vi "Check_Single_Box_move.vi"(3 "Traverse Name":string, 5 "Exclude Array":T3[](array[typedef])=[{"Sizes"=[{"Max"=15000.0, "Min"=0.0}, {"Max"=1000.0, "Min"=-1000.0}, {"Max"=300.0, "Min"=0.0}], "Name"="Roughness Elements", "Exclude Type"=enum."Allow only vertical moves"}, {"Sizes"=[{"Max"=17000.0, "Min"=16000.0}, {"Max"=200.0, "Min"=-200.0}, {"Max"=-50.0, "Min"=-250.0}], "Name"="B204", "Exclude Type"=enum."Exclude completely"}] {"Sizes"."Min" format="%#.1f"; "Sizes"."Max" format="%#.1f"}, 6 "Volume":T2=[{"Max"=15001.0, "Min"=12000.0}, {"Max"=1000.0, "Min"=-1000.0}, {"Max"=700.0, "Min"=0.0}] {"Min" format="%#.1f"; "Max" format="%#.1f"}, 8 "New Position":sgl[](array[numeric])=[0.0, 0.0, 0.0] format="%.2f", 9 "Current position":sgl[](array[numeric])=[0.0, 0.0, 0.0] format="%.2f") -> (0 "Error Comments":string, 2 "Position At Crash":dbl[](array[numeric]) format="%.2f")   [LabVIEW 2018]
uses:
  Exclude_cluster.ctl
  Box_size.ctl
  Exclusion_type.ctl
  Moving Axis.ctl
  Globals/Trav_pos_global.vi
panel:
  in  "Traverse active parts":T1
  out "Numeric":i32
  # "X                Y                   Z"
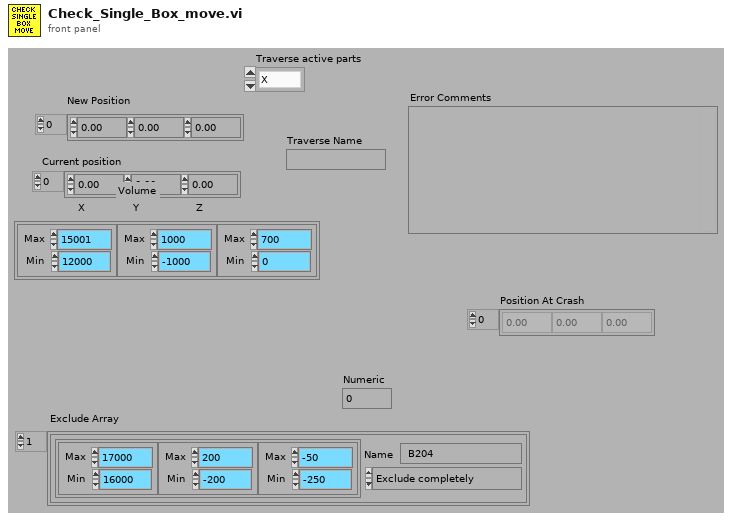
[diagram p1: front panel]
types:
  T1 = typedef "Moving Axis.ctl" = enum16{"X", "XY", "XYZ"}
  T2 = typedef "Box_size.ctl" = cluster{"Max":sgl, "Min":sgl}[]
  T3 = typedef "Exclude_cluster.ctl" = cluster{"Sizes":T2, "Name":string, "Exclude Type":T4}
  T4 = typedef "Exclusion_type.ctl" = enum16{"Exclude completely", "Allow only vertical moves"}
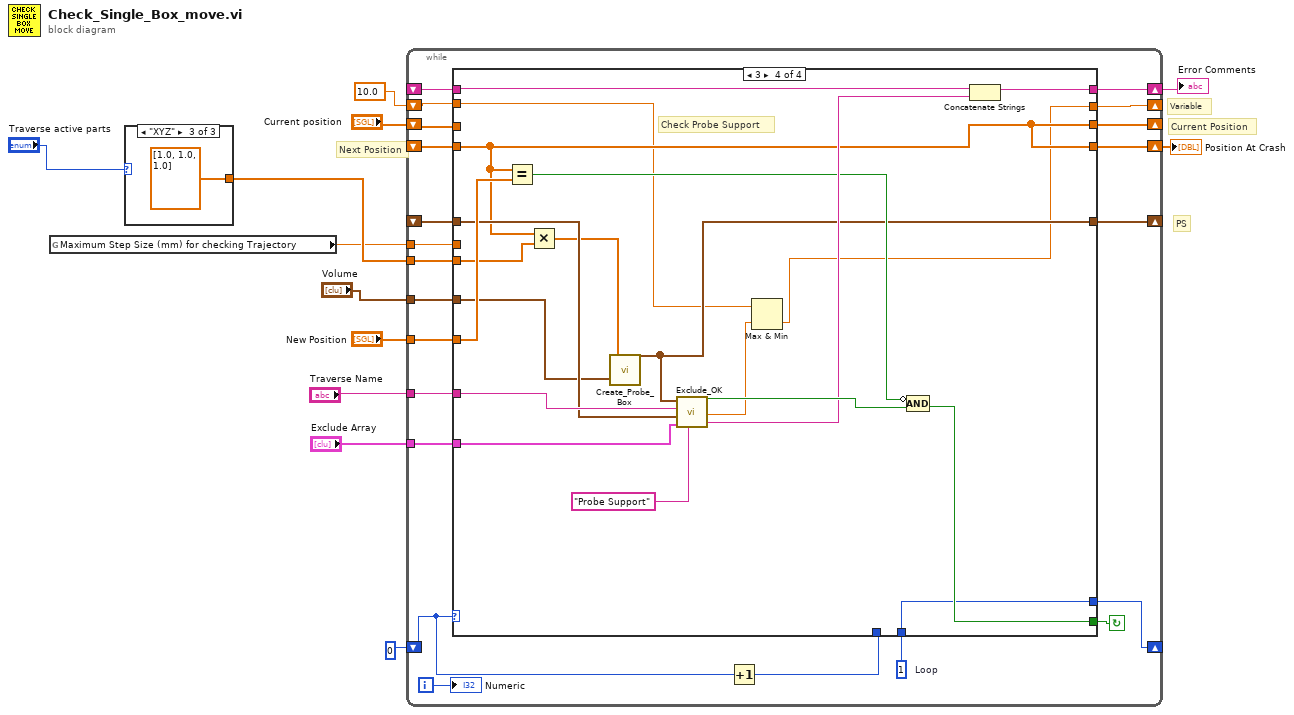
[diagram p0: block diagram]
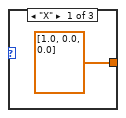
[diagram p2: hidden frame]
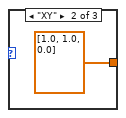
[diagram p3: hidden frame]
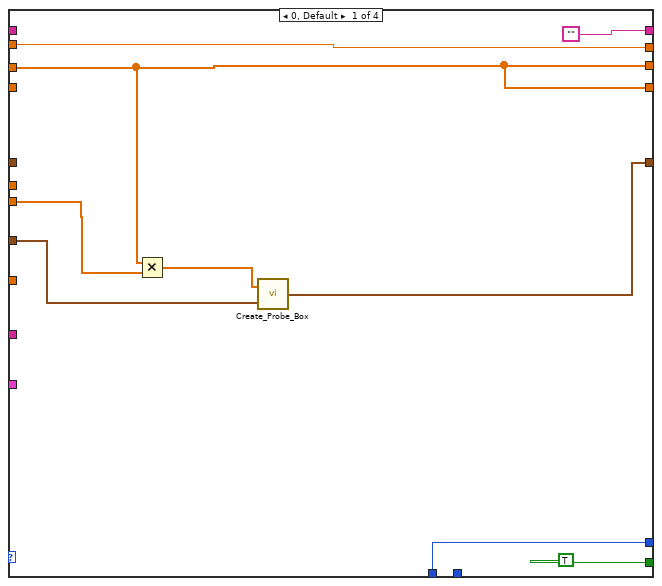
[diagram p4: hidden frame]
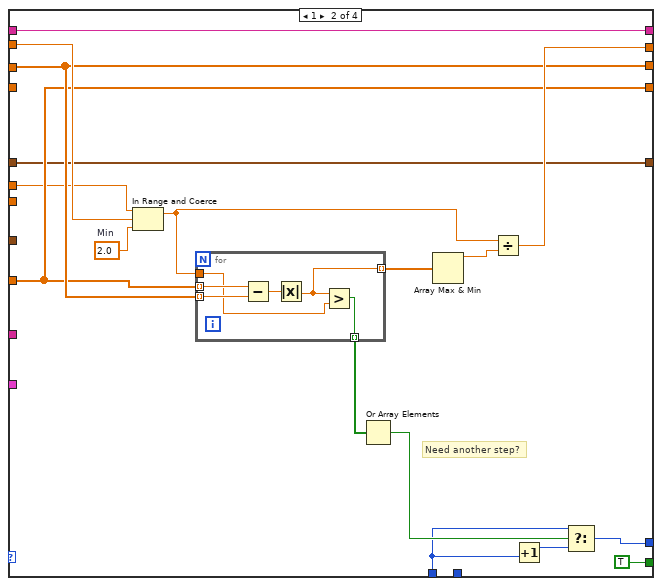
[diagram p5: hidden frame]
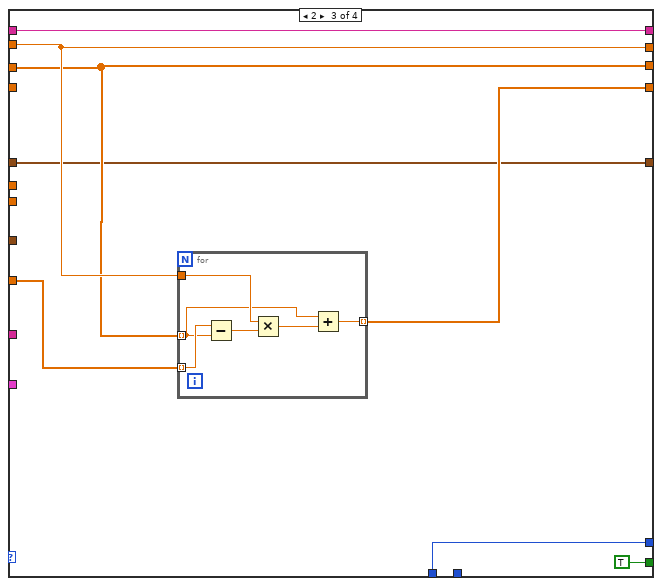
[diagram p6: hidden frame]
diagram:
  # "PS"
  # "Current Position"
  # "Next Position"
  # "Variable"
  n1 = global read "Trav_pos_global.vi" "Maximum Step Size (mm) for checking Trajectory"() -> (w2:sgl)
  n2 = case shown="\"XYZ\"" "Traverse active parts" {
    tunnel: [sgl[] [1.0, 0.0, 0.0] ("Current position") sgl[] [1.0, 1.0, 0.0] ("Current position") sgl[] [1.0, 1.0, 1.0] ("Current position")] -> w3
    frame "X" {
    }
    frame "XY" {
    }
    frame "XYZ" {
    }
  }
  n3 = while {
    tunnel: "New Position" -> [w23]
    shift-left: _ -> [w25]
    shift-right: [w26] -> w8
    shift-left: 0 -> [w29]
    shift-right: [w28] -> _
    tunnel: "Traverse Name" -> [w30]
    tunnel: "Exclude Array" -> [w32]
    shift-left: sgl 10.0 ("Separation Distance") -> [w36]
    shift-right: [w31] -> _
    shift-left: _ -> [w24]
    shift-right: [w34] -> w6
    shift-left: "Current position" -> [w37]
    shift-right: [w35] -> _
    shift-right: [w19] -> _
    shift-left: _ -> [w18]
    tunnel: "Volume" -> [w20]
    tunnel: w3 -> [w17]
    tunnel: w2 -> [w16]
    i -> [w21]
    stop <- w33 continue-if-true
    w22 = 1  # Loop
    n4 = Increment(x=w29) -> (x+1=w27:i32)
    n5 = case shown="3" w29 {
      tunnel: w37 -> [w40 w51 w74 _]
      tunnel: w36 -> [w46 w63 w75 w86]
      tunnel: [w40 w51 w74 w91] -> w35
      tunnel: [w40 w50 w73 w91] -> w34
      tunnel: [TRUE ("Box Inside") TRUE ("Box Inside") TRUE ("Box Inside") w95] -> w33
      tunnel: w32 -> [_ _ _ w103]
      tunnel: [w46 w56 w75 w84] -> w31
      tunnel: w30 -> [_ _ _ w102]
      tunnel: [w38 w54 w71 w94] -> w28
      tunnel: w27 -> [w38 w52 w71 _]
      tunnel: ["" w61 w77 w99] -> w26
      tunnel: w25 -> [_ w61 w77 w100]
      tunnel: w24 -> [_ _ _ w91]
      tunnel: w23 -> [_ w50 w72 w97]
      tunnel: w22 -> [_ _ _ w94]
      tunnel: w20 -> [w43 _ _ w92]
      tunnel: [w42 w48 w70 w88] -> w19
      tunnel: w18 -> [_ w48 w70 w93]
      tunnel: w17 -> [w41 _ _ w90]
      tunnel: w16 -> [_ w47 _ _]
      frame 0, Default {
        n6 = Multiply(x=w40, y=w41) -> (x*y=w39:sgl[])
        n7 = call "Create_Probe_Box.vi"("Probe Volume"=w43, "Probe Position"=w39) -> ("Current Probe Volume"=w42:T2)
      }
      frame 1 {
        w59 = sgl 2.0  # Min
        # "Need another step?"
        n8 = In Range and Coerce(upper limit=w47, x=w63, lower limit=w59) -> (coerced(x)=w49:sgl)  [unwired: 1 out]
        n9 = for {
          tunnel: w50 -> [w69] mode=indexing
          tunnel: w51 -> [w68] mode=indexing
          tunnel: w49 -> [w67]
          tunnel: [w65] -> w60 mode=indexing
          tunnel: [w64] -> w58 mode=indexing
          n10 = Subtract(x=w69, y=w68) -> (x-y=w66:sgl)
          n11 = Absolute Value(x=w66) -> (abs(x)=w64:sgl)
          n12 = Greater?(x=w64, y=w67) -> (0:w65:bool)
        }
        n13 = Or Array Elements(Boolean array=w60) -> (logical OR=w55:bool)
        n14 = Array Max & Min(array=w58) -> (max value=w57:sgl)  [unwired: 3 out]
        n15 = Divide(x=w49, y=w57) -> (x/y=w56:sgl)
        n16 = Increment(x=w52) -> (x+1=w53:i32)
        n17 = Select(t=w52, s=w55, f=w53) -> (s? t:f=w54:i32)
      }
      frame 2 {
        n18 = for {
          tunnel: w72 -> [w83] mode=indexing
          tunnel: w74 -> [w79] mode=indexing
          tunnel: w75 -> [w81]
          tunnel: [w78] -> w73 mode=indexing
          n19 = Subtract(x=w83, y=w79) -> (x-y=w82:sgl)
          n20 = Multiply(x=w81, y=w82) -> (x*y=w80:sgl)
          n21 = Add(x=w79, y=w80) -> (x+y=w78:sgl)
        }
      }
      frame 3 {
        # "Check Probe Support"
        n22 = Equal?(x=w91, y=w97) -> (x = y?=w96:bool)
        n23 = Multiply(x=w91, y=w90) -> (x*y=w89:sgl[])
        n24 = call "Create_Probe_Box.vi"("Probe Volume"=w92, "Probe Position"=w89) -> ("Current Probe Volume"=w88:T2)
        n25 = call "Exclude_OK.vi"("Probe Volume"=w88, "Traverse Name"=w102, "Previous Probe Volume"=w93, "Exclude Array"=w103, "Volume Name"="Probe Support") -> ("Probe OK?"=w101:bool, "Separation Distance"=w85:sgl, "Error Comments"=w98:string)
        n26 = Max & Min(x=w86, y=w85) -> (min(x,y)=w84:sgl)  [unwired: 1 out]
        n27 = Compound Arithmetic op=AND(invert w96, w101) -> (w95:bool)
        n28 = Concatenate Strings(w100, w98) -> (w99:string)
      }
    }
    "Numeric" <- w21
  }
  "Error Comments" <- w8
  "Position At Crash" <- w6
